vi "KEB VF status global.vi"() -> ()   [LabVIEW 2019]
panel:
  in  "KEB V/F status":bool
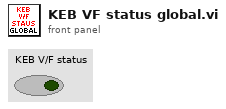
[diagram p1: front panel]
diagram:
